vi "Clamp Vertical Max VI.vi"(0 "Image":T2, 2 "Rectangle":T5 {"Rotation" format="%.2f"; "Left" scale=0.0..1024.0; "Right" scale=0.0..1024.0}, 3 "Coordinate System":T4 {"Measurement System"."Axis Reference" items=["Direct", "Indirect"]; "Measurement System"."Angle (deg)" format="%.2f"; "Measurement System"."Origin"."Y" format="%.2f"; "Measurement System"."Origin"."X" format="%.2f"; "Reference System"."Axis Reference" items=["Direct", "Indirect"]; "Reference System"."Angle (deg)" format="%.2f"; "Reference System"."Origin"."Y" format="%.2f"; "Reference System"."Origin"."X" format="%.2f"}, 5 "error in (no error)":errorcluster, 8 "Settings":T3={"Contrast"=40, "Filter width"=4, "Steepness"=2, "Subsampling Ratio"=5, "Show Search Area"=FALSE, "Show Search Lines"=FALSE, "Show Edges Found"=FALSE, "Show Result"=TRUE}) -> (7 "Line Coordinates":T1(array[cluster]) {"?"."Y" format="%.2f"; "?"."X" format="%.2f"; "?"."Y" format="%.2f"; "?"."X" format="%.2f"}, 9 "appended array":cluster{"X":sgl, "Y":sgl}[](array[cluster]), 10 "Edge Coordinates":cluster{"X":sgl, "Y":sgl}[](array[cluster]) {"Y" format="%.2f"; "X" format="%.2f"}, 11 "Perpendicular Lines":T1(array[cluster])=[{{"X"=55.0, "Y"=48.0}, {"X"=263.0, "Y"=104.0}}, {{"X"=53.0, "Y"=53.0}, {"X"=262.0, "Y"=109.0}}, {{"X"=52.0, "Y"=58.0}, {"X"=261.0, "Y"=113.0}}, {{"X"=51.0, "Y"=62.0}, {"X"=259.0, "Y"=118.0}}, {{"X"=49.0, "Y"=67.0}, {"X"=258.0, "Y"=123.0}}, {{"X"=48.0, "Y"=72.0}, {"X"=257.0, "Y"=128.0}}, {{"X"=47.0, "Y"=77.0}, {"X"=255.0, "Y"=133.0}}, {{"X"=46.0, "Y"=82.0}, {"X"=254.0, "Y"=138.0}}, {{"X"=44.0, "Y"=87.0}, {"X"=253.0, "Y"=142.0}}, {{"X"=43.0, "Y"=91.0}, {"X"=252.0, "Y"=147.0}}, {{"X"=42.0, "Y"=96.0}, {"X"=250.0, "Y"=152.0}}] {"?"."Y" format="%.2f"; "?"."X" format="%.2f"; "?"."Y" format="%.2f"; "?"."X" format="%.2f"}, 13 "Points":cluster{"X":sgl, "Y":sgl}[](array[cluster])=[{"X"=67.0, "Y"=51.0}, {"X"=230.0, "Y"=95.0}, {"X"=66.0, "Y"=56.0}, {"X"=230.0, "Y"=100.0}, {"X"=66.0, "Y"=62.0}, {"X"=230.0, "Y"=105.0}, {"X"=66.0, "Y"=66.0}, {"X"=230.0, "Y"=110.0}, {"X"=65.0, "Y"=71.0}, {"X"=230.0, "Y"=115.0}, {"X"=65.0, "Y"=77.0}, {"X"=230.0, "Y"=121.0}, {"X"=65.0, "Y"=82.0}, {"X"=229.0, "Y"=126.0}, {"X"=65.0, "Y"=87.0}, {"X"=229.0, "Y"=131.0}, {"X"=64.0, "Y"=92.0}, {"X"=229.0, "Y"=136.0}, {"X"=64.0, "Y"=97.0}, {"X"=229.0, "Y"=141.0}, {"X"=64.0, "Y"=102.0}, {"X"=229.0, "Y"=146.0}] {"Y" format="%.2f"; "X" format="%.2f"}, 14 "Image Out":T2, 16 "Distance":sgl format="%.2f", 17 "Coordinate System (duplicate)":T4 {"Measurement System"."Axis Reference" items=["Direct", "Indirect"]; "Measurement System"."Angle (deg)" format="%.2f"; "Measurement System"."Origin"."Y" format="%.2f"; "Measurement System"."Origin"."X" format="%.2f"; "Reference System"."Axis Reference" items=["Direct", "Indirect"]; "Reference System"."Angle (deg)" format="%.2f"; "Reference System"."Origin"."Y" format="%.2f"; "Reference System"."Origin"."X" format="%.2f"}, 19 "error out":errorcluster)   [LabVIEW 2019]
uses:
  <vilib>/vision/Image Controls.llb/IMAQ Image.ctl
  <vilib>/vision/NI_Vision_Development_Module.lvlib
panel:
  out "Elapsed time (ms)":u32
  # "Start Point"
  # "End Point"
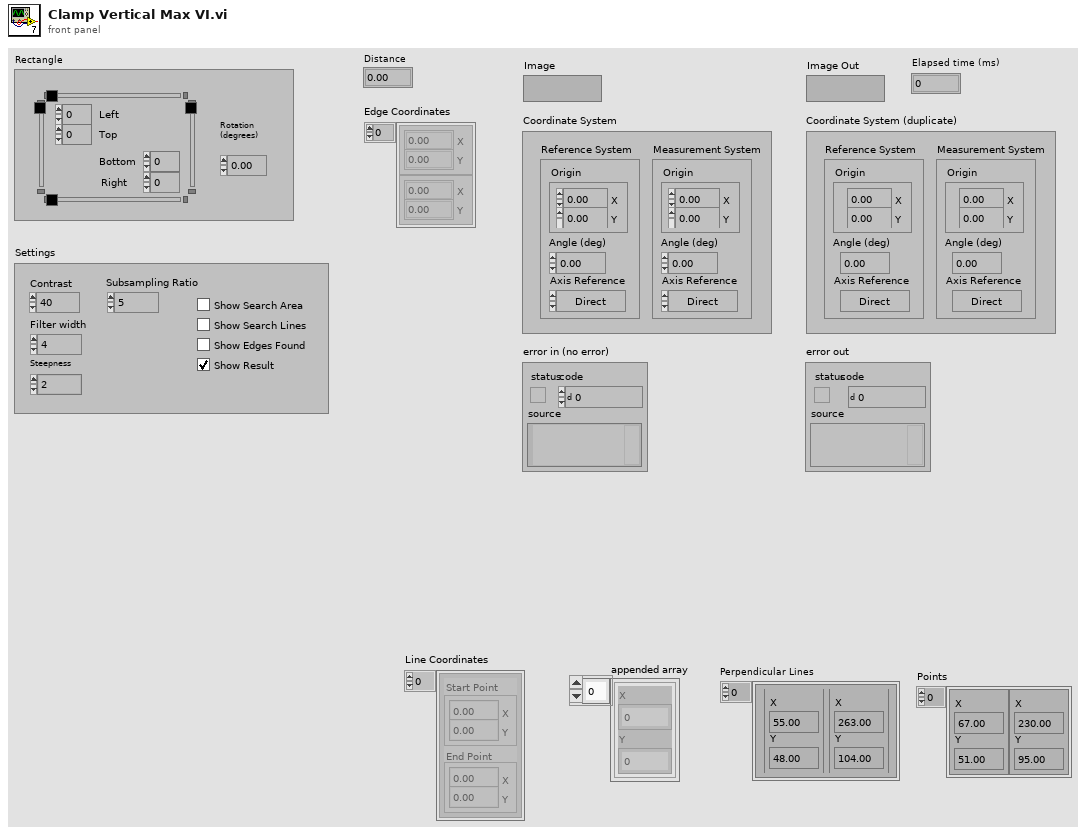
[diagram p1: front panel]
types:
  T1 = cluster{cluster{"X":sgl, "Y":sgl}, cluster{"X":sgl, "Y":sgl}}[]
  T2 = typedef "IMAQ Image.ctl" = refnum<image>
  T3 = cluster{"Contrast":i32, "Filter width":i32, "Steepness":i32, "Subsampling Ratio":u32, "Show Search Area":bool, "Show Search Lines":bool, "Show Edges Found":bool, "Show Result":bool}
  T4 = typedef "IMAQ Coordinate System" = cluster{"Reference System":cluster{"Origin":cluster{"X":sgl, "Y":sgl}, "Angle (deg)":sgl, "Axis Reference":u32}, "Measurement System":cluster{"Origin":cluster{"X":sgl, "Y":sgl}, "Angle (deg)":sgl, "Axis Reference":u32}}
  T5 = typedef "IMAQ Rectangle" = cluster{"Left":i32, "Top":i32, "Right":i32, "Bottom":i32, "Rotation":dbl}
  T6 = cluster{"Interpolation Type":enum32{"", "Quadratic", "Cubic Spline"}, "SubPixel Accuracy":enum32{"None", "One Half", "One Third", "One Fourth", "One Fifth", "One Sixth", "One Seventh", "One Eight", "One Ninth", "One Tenth", "One Eleventh", "One Twelveth"}}
  T7 = enum32{"Get First Edge", "Get First + Last Edge", "Get All Edges"}
  T8 = cluster{"Origin":cluster{"X":sgl, "Y":sgl}, "Angle (deg)":sgl, "Axis Reference":u32}
  T9 = typedef "ROI Descriptor" = cluster{"Global Rectangle":i32[], "Contours":cluster{"ID":enum32{"External", "Internal"}, "Type":u32, "Coordinates":i32[]}[]}
  T10 = cluster{"Contrast":i32, "Filter width":i32, "Steepness":i32}
  T11 = cluster{"Show Search Area":bool, "Show Search Lines":bool, "Show Edges Found":bool, "Show Result":bool}
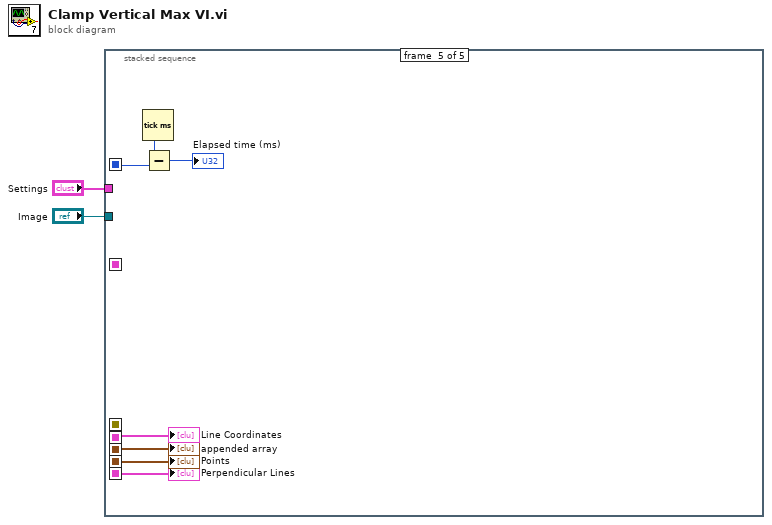
[diagram p0: block diagram]
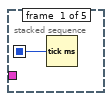
[diagram p2: hidden frame]
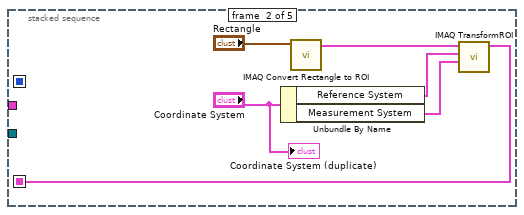
[diagram p3: hidden frame]
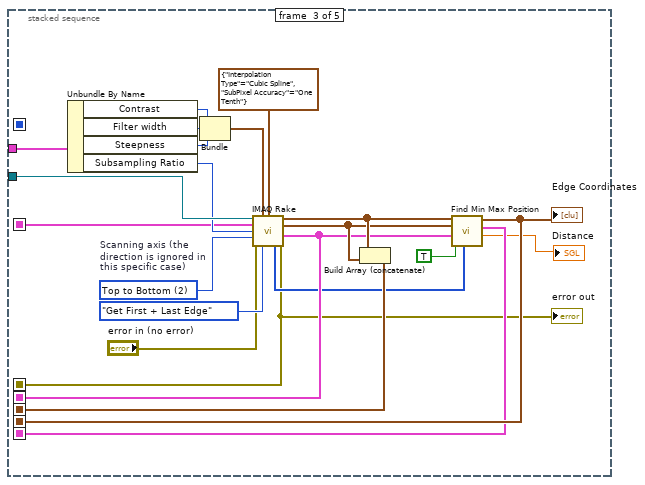
[diagram p4: hidden frame]
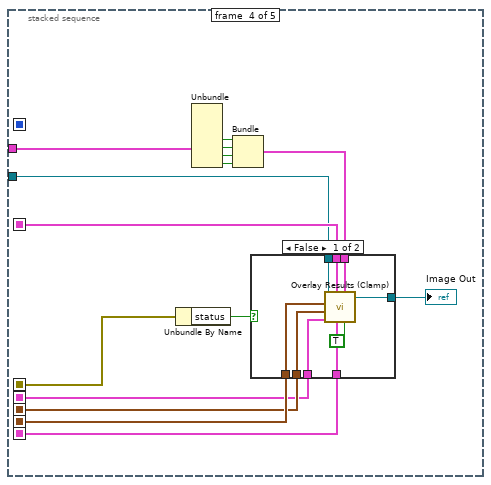
[diagram p5: hidden frame]
diagram:
  n1 = stacked-sequence {
    seq-local: [_ _ w19 _ _] -> [_ _ _ w46 w58]
    seq-local: [w3 _ _ _ _] -> [_ _ _ _ w63]
    seq-local: [_ _ w20 _ _] -> [_ _ _ w45 w59]
    seq-local: [_ _ w21 _ _] -> [_ _ _ w44 w60]
    seq-local: [_ _ w18 _ _] -> [_ _ _ w38 w57]
    seq-local: [_ w7 _ _ _] -> [_ _ w12 w36 _]
    seq-local: [_ _ w10 _ _] -> [_ _ _ w33 _]
    tunnel: "Settings" -> [_ _ w23 w39 _]
    tunnel: "Image" -> [_ _ w24 w35 _]
    frame #0 {
      n2 = Tick Count (ms)() -> (millisecond timer value=w3:u32)
    }
    frame #1 {
      n3 = Unbundle By Name("Coordinate System") -> ("Reference System"=w5:T8, "Measurement System"=w4:T8)
      n4 = call "IMAQ Convert Rectangle to ROI"("Rectangle"="Rectangle") -> ("ROI Descriptor"=w9:T9)  [unwired: 1 in, 8 out]
      n5 = call "IMAQ TransformROI"("New Reference"=w4, "Base Reference"=w5, "ROI Descriptor"=w9) -> ("ROI Descriptor out"=w7:T9)  [unwired: 1 in, 7 out]
      "Coordinate System (duplicate)" <- "Coordinate System"
    }
    frame #2 {
      w27 = u32 2 items=["Left to Right", "Right to Left", "Top to Bottom", "Bottom to Top"]  # Scanning axis (the direction is ignored in this specific case)
      # "Find Edges"
      n6 = Unbundle By Name(w23) -> ("Contrast"=w15:i32, "Filter width"=w16:i32, "Steepness"=w14:i32, "Subsampling Ratio"=w13:u32)
      n7 = Bundle("Contrast"=w15, "Filter width"=w16, "Steepness"=w14) -> (w31:T10)  [unwired: 1 out]
      n8 = call "IMAQ Rake"("Image"=w24, "Edge Parameters"=w31, "SubPixel Information"=T6 {"Interpolation Type"=enum."Cubic Spline", "SubPixel Accuracy"=enum."One Tenth"}, "ROI Descriptor"=w12, "Step Size"=w13, "Scan Direction"=w27, "error in (no error)"="error in (no error)", "Process"=T7."Get First + Last Edge") -> ("First Edges"=w26:cluster{"X":sgl, "Y":sgl}[], "Last Edges"=w25:cluster{"X":sgl, "Y":sgl}[], "Line Coordinates"=w21:T1, "Lines with Edges"=w11:u32[], "error out"=w10:errorcluster)  [unwired: 1 in, 2 out]
      "error out" <- w10
      n9 = Build Array (concatenate)(w26, w25) -> (w20:cluster{"X":sgl, "Y":sgl}[])
      n10 = call <vilib>:"Find Min Max Position.vi"("Lines with Edges (first)"=w11, "Min / Max"=TRUE, "Search Lines"=w21, "Last Edges"=w25, "First Edges"=w26) -> ("Distance"=→"Distance":sgl, "Perpendicular Lines"=w18:T1, "Points"=w19:cluster{"X":sgl, "Y":sgl}[])  [unwired: 1 in, 3 out]
      "Edge Coordinates" <- w19
    }
    frame #3 {
      # "Update Overlay"
      n11 = Unbundle By Name(w33) -> ("status"=w32:bool)
      n12 = Unbundle(w39) -> ("Show Search Area"=w43:bool, "Show Search Lines"=w42:bool, "Show Edges Found"=w41:bool, "Show Result"=w40:bool)  [unwired: 4 out]
      n13 = Bundle("Show Search Area"=w43, "Show Search Lines"=w42, "Show Edges Found"=w41, "Show Result"=w40) -> (w37:T11)  [unwired: 1 out]
      n14 = case shown="False" w32 {
        tunnel: w46 -> [w55 _]
        tunnel: w45 -> [w54 _]
        tunnel: w44 -> [w53 _]
        tunnel: w38 -> [w52 _]
        tunnel: w37 -> [w50 _]
        tunnel: w36 -> [w49 _]
        tunnel: w35 -> [w48 w56]
        tunnel: [w47 w56] -> w34
        frame False {
          n15 = call <vilib>:"Overlay Results (Clamp).vi"("Min / Max"=TRUE, "Setup"=w50, "Perpendicular Lines"=w52, "ROI Descriptor"=w49, "Search Lines"=w53, "All Edges Found"=w54, "Measurement Edges"=w55, "Image In"=w48) -> ("Image Out"=w47:T2)  [unwired: 3 out]
        }
        frame True {
        }
      }
      "Image Out" <- w34
    }
    frame #4 {
      n16 = Tick Count (ms)() -> (millisecond timer value=w62:u32)
      n17 = Subtract(x=w62, y=w63) -> (x-y=→"Elapsed time (ms)":u32)
      "Line Coordinates" <- w60
      "appended array" <- w59
      "Points" <- w58
      "Perpendicular Lines" <- w57
    }
  }
